vi "getTableRowCount.vi"(8 "error in (no error)":errorcluster, 11 "Table":refnum<k24>) -> (0 "error out":errorcluster, 2 "Count":i32, 3 "Table":refnum<k24>)   [LabVIEW 2017, in "LabVIEW NPOI.lvlib" / "xwpfReader.lvclass"]
uses:
  xwpfReader.lvclass
  C:/Users/Neo/Desktop/Dev_Tools_BR/LabVIEW_NPOI/lib/NPOI 2.1.1/NPOI.OOXML.dll
  lib/NPOI 2.1.1/NPOI.OOXML.dll
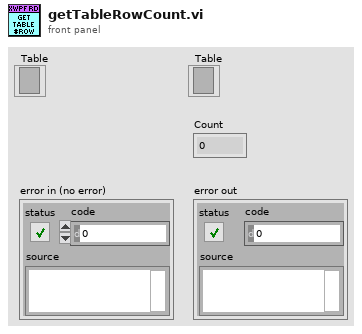
[diagram p1: front panel]
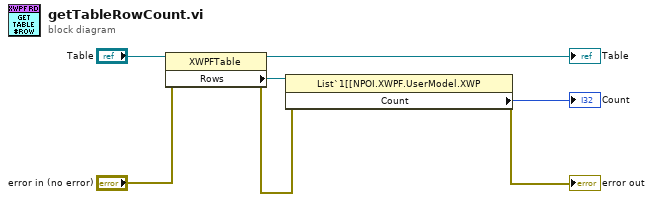
[diagram p0: block diagram]
diagram:
  n1 = property class="XWPFTable"(reference="Table", error in="error in (no error)") -> (reference out=→"Table":refnum<k24>, error out=w6:errorcluster, "Rows"=w3:refnum<k24>)
  n2 = property class="List`1[[NPOI.XWPF.UserModel.XWP"(reference=w3, error in=w6) -> (error out=→"error out":errorcluster, "Count"=→"Count":i32)  [unwired: 1 out]
